vi "PH_Init.vi"() -> (0 "PH_Init_Data":T1)   [LabVIEW 2019]
panel:
  out "Calib Error":bool
  out "Status":string
  out "Initialization Error":bool
  out "DLL Version":string
  out "Initialization Status":string
  out "Deviceindex":i32
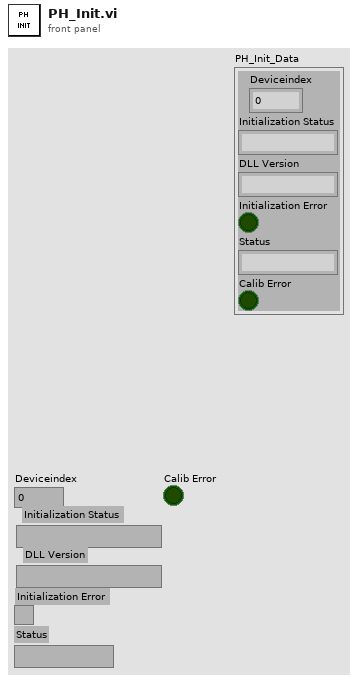
[diagram p1: front panel]
types:
  T1 = cluster{"Deviceindex":i32, "Initialization Status":string, "DLL Version":string, "Initialization Error":bool, "Status":string, "Calib Error":bool}
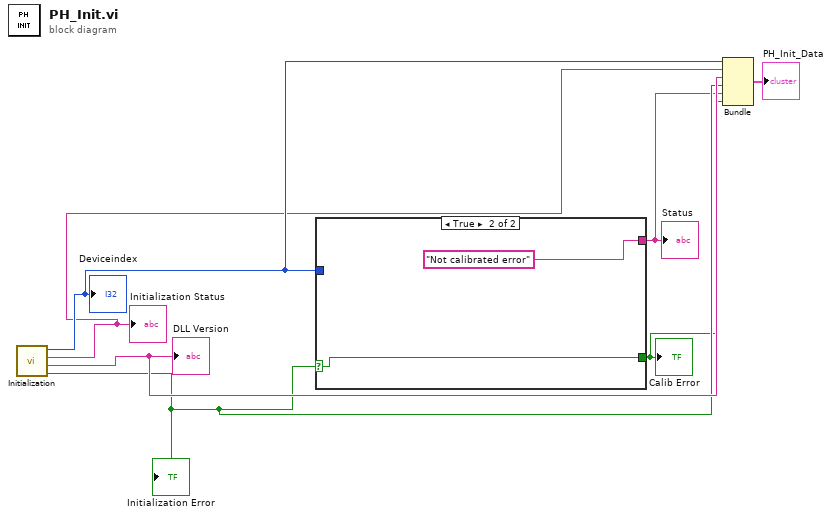
[diagram p0: block diagram]
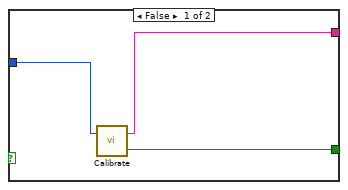
[diagram p2: hidden frame]
diagram:
  n1 = call "Initialization.vi"() -> ("Deviceindex"=w7:i32, "Initialization Status"=w6:string, "DLL Version"=w5:string, "Initialization Error"=w4:bool)  [unwired: 2 in]
  "Deviceindex" <- w7
  "Initialization Status" <- w6
  "DLL Version" <- w5
  "Initialization Error" <- w4
  n2 = case shown="True" w4 {
    selector: w4 -> [_ w11]
    tunnel: w7 -> [w10 _]
    tunnel: [w9 "Not calibrated error"] -> w3
    tunnel: [w8 w11] -> w2
    frame False {
      n3 = call "Calibrate.vi"("Deviceindex"=w10) -> ("Calib Error"=w8:bool, "Status"=w9:string)  [unwired: 1 in]
    }
    frame True {
    }
  }
  "Status" <- w3
  "Calib Error" <- w2
  n4 = Bundle("Deviceindex"=w7, "Initialization Status"=w6, "DLL Version"=w5, "Initialization Error"=w4, "Status"=w3, "Calib Error"=w2) -> (→"PH_Init_Data":T1)  [unwired: 1 in]
